vi "FB_MFA_Read_Halls1.vi"() -> (3 "Hall Get":i16)   [LabVIEW 2011]
panel:
  out "error Hall Get":errorcluster
  out "AAABuild":i32
  in  "MintController":refnum<k7>(container)
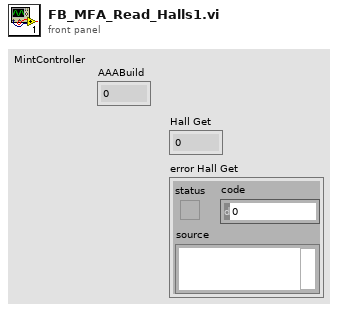
[diagram p1: front panel]
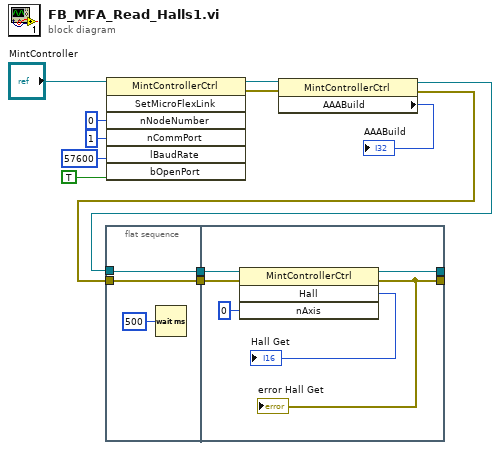
[diagram p0: block diagram]
diagram:
  n1 = flat-sequence {
    tunnel: w4 -> [w14]
    tunnel: [w14] -> w3
    tunnel: w2 -> [w13]
    tunnel: [w13] -> w1
    tunnel: [w19] -> _
    tunnel: [w18] -> _
    tunnel: w3 -> [w17]
    tunnel: w1 -> [w16]
    frame #0 {
      n2 = Wait (ms)(milliseconds to wait=u32 500) -> ()  [unwired: 1 out]
    }
    frame #1 {
      n3 = invoke class="MintControllerCtrl" method="Hall"(reference=w17, error in=w16, "nAxis"=i16 0 ("nBank")) -> (reference out=w19:refnum<k7>, error out=w18:errorcluster, "Hall"=→"Hall Get":i16)  [unwired: 1 in, 1 out]
      "error Hall Get" <- w18
    }
  }
  n4 = invoke class="MintControllerCtrl" method="SetMicroFlexLink"(reference="MintController", "nNodeNumber"=i16 0, "nCommPort"=i16 1, "lBaudRate"=57600, "bOpenPort"=TRUE) -> (reference out=w12:refnum<k7>, error out=w6:errorcluster)  [unwired: 2 in, 5 out]
  n5 = property class="MintControllerCtrl"(reference=w12, error in=w6) -> (reference out=w4:refnum<k7>, error out=w2:errorcluster, "AAABuild"=→"AAABuild":i32)
